vi "Ring-Add Filename.vi"(0 "Ring in":refnum<vi>, 7 "filename":string) -> ()   [LabVIEW 2015]
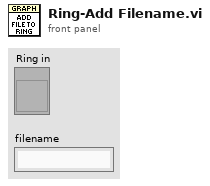
[diagram p1: front panel]
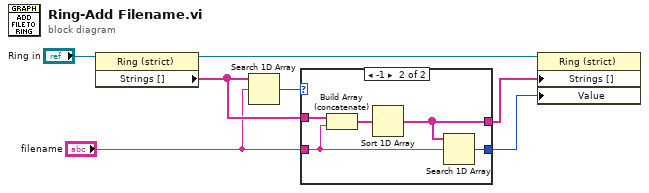
[diagram p0: block diagram]
diagram:
  n1 = property on="Property Node" class="Ring (strict)"(reference="Ring in") -> (reference out=w6:refnum<vi>, "Strings []"=w4:string[])  [unwired: 1 in, 1 out]
  n2 = Search 1D Array(1D array=w4, element="filename") -> (index of element=w5:i32)  [unwired: 1 in]
  n3 = case shown="-1" w5 {
    selector: w5 -> [w8 _]
    tunnel: [w9 w12] -> w3
    tunnel: "filename" -> [_ w11]
    tunnel: w4 -> [w9 w13]
    tunnel: [w8 w10] -> w1
    frame 0, Default {
    }
    frame -1 {
      n4 = Build Array (concatenate)(w13, w11) -> (w14:string[])
      n5 = Sort 1D Array(array=w14) -> (sorted array=w12:string[])
      n6 = Search 1D Array(1D array=w12, element=w11) -> (index of element=w10:i32)  [unwired: 1 in]
    }
  }
  n7 = property on="Property Node" class="Ring (strict)"(reference=w6, "Strings []"=w3, "Value"=w1) -> ()  [unwired: 1 in, 2 out]
